vi "Waveform, Write to New File.vi"(5 "filepath":path, 6 "error in":errorcluster, 8 "prc waveform":waveform(dbl)={"t0"=timestamp(0 s since 1904-01-01), "dt"=1e-05, "Y"=[]}, 9 "raw waveform":waveform(dbl)={"t0"=timestamp(0 s since 1904-01-01), "dt"=1e-05, "Y"=[]}) -> (0 "error out":errorcluster, 2 "prc waveform dup":waveform(dbl)={"t0"=timestamp(0 s since 1904-01-01), "dt"=nan, "Y"=[]}, 3 "raw waveform out":waveform(dbl)={"t0"=timestamp(0 s since 1904-01-01), "dt"=nan, "Y"=[]}, 4 "file saved":bool)   [LabVIEW 2010]
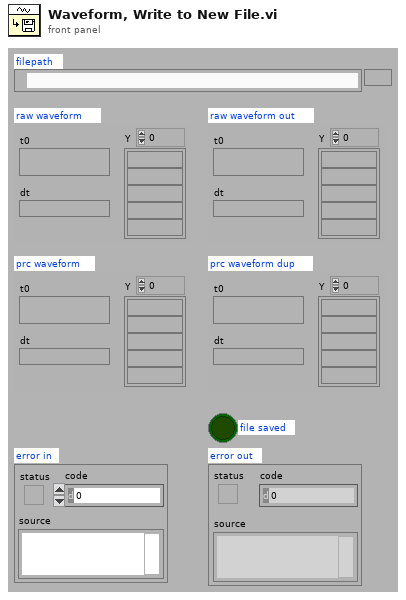
[diagram p1: front panel]
types:
  T1 = enum16{"open", "replace", "create", "open or create", "replace or create", "replace or create with confirmation"}
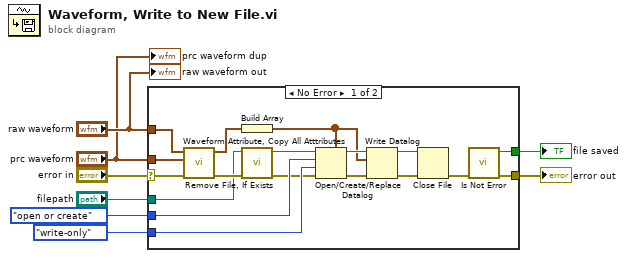
[diagram p0: block diagram]
diagram:
  n1 = case shown="No Error" "error in" {
    selector: "error in" -> [w14 w27]
    tunnel: "filepath" -> [w10 _]
    tunnel: [w16 w27] -> w7
    tunnel: T1."open or create" ("operation (0:open)") -> [w22 _]
    tunnel: enum16{"read/write", "read-only", "write-only"}."write-only" ("access (0:read/write)") -> [w21 _]
    tunnel: "prc waveform" -> [w9 _]
    tunnel: [w15 _] -> w3
    tunnel: "raw waveform" -> [w12 _]
    frame No Error {
      n2 = call "Waveform Attribute, Copy All Atttributes.vi"("error in"=w14, "src waveform"=w9, "dst waveform"=w12) -> ("error out"=w13:errorcluster, "dst waveform out"=w11:waveform(dbl))  [unwired: 3 in, 2 out]
      n3 = Build Array "Build Array"(w11) -> (w18:waveform(dbl)[])
      n4 = call "Remove File, If Exists.vi"("error in"=w13, "filepath"=w10) -> ("error out"=w20:errorcluster, "filepath dup"=w19:path)  [unwired: 4 in]
      n5 = Open/Create/Replace Datalog(5:w18, 8:w20, 9:w21, 10:w22, 11:w19) -> (0:w26:errorcluster, 3:w23:refnum<k1>)  [unwired: 1 in, 1 out]
      n6 = Write Datalog(4:w26, 6:w18, 7:w23) -> (0:w25:errorcluster, 3:w24:refnum<k1>)
      n7 = Close File(refnum=w24, error in=w25) -> (error out=w17:errorcluster)  [unwired: 1 out]
      n8 = call "Is Not Error.vi"("error in"=w17) -> ("error out"=w16:errorcluster, "!error"=w15:bool)  [unwired: 5 in, 1 out]
    }
    frame Error {
    }
  }
  "error out" <- w7
  "file saved" <- w3
  "raw waveform out" <- "raw waveform"
  "prc waveform dup" <- "prc waveform"
